vi "UART Write.vi"() -> ()   [LabVIEW 2023, in "CTI-Visa-Scratchpad.lvlib"]
uses:
  CTI-Visa-Scratchpad.lvlib
  CTI-Visa/CTI-Visa.lvlib
panel:
  in  "RX GPIO":u8=1
  in  "TX GPIO":u8
  in  "Baud":u32=19200
  in  "UART":u8
  in  "Write":bool
  in  "Data":string="Hello, world!"
  in  "stop":bool
  in  "Port":refnum<visa-resource-name>="COM3"
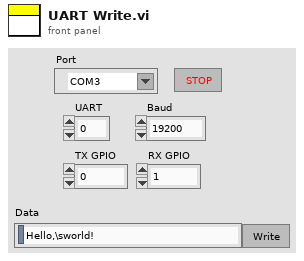
[diagram p1: front panel]
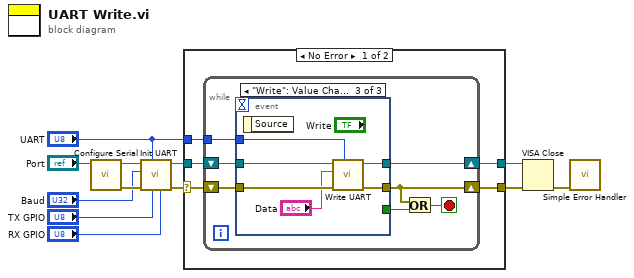
[diagram p0: block diagram]
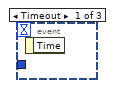
[diagram p2: hidden frame]
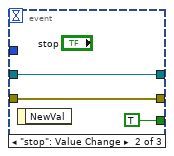
[diagram p3: hidden frame]
diagram:
  n1 = call "Configure Serial.vi"("VISA resource name in"="Port") -> ("error out"=w10:errorcluster, "VISA resource name"=w11:refnum<visa-resource-name>)  [unwired: 9 in]
  n2 = call "Init UART.vi"("RX GPIO"="RX GPIO", "TX GPIO"="TX GPIO", "UART"="UART", "error in (no error)"=w10, "Baud"="Baud", "VISA resource name in"=w11) -> ("error out"=w9:errorcluster, "VISA resource name"=w8:refnum<visa-resource-name>)  [unwired: 4 in]
  n3 = case shown="No Error" w9 {
    selector: w9 -> [w15 w35]
    tunnel: w8 -> [w16 w34]
    tunnel: "UART" -> [w17 _]
    tunnel: [w14 w35] -> w7
    tunnel: [w13 w34] -> w6
    frame No Error {
      n4 = while {
        tunnel: w17 -> [w23]
        shift-right: [w22] -> w13
        shift-left: w16 -> [w24]
        shift-right: [w20] -> w14
        shift-left: w15 -> [w21]
        stop <- w18 stop-if-true
        n5 = event shown="[2] \"Write\": Value Change" {
          selector: _ -> [_ _ _]
          dyn-events: _ -> [_ _ _]
          timeout: _ -> [_ _ _]
          tunnel: w24 -> [_ w27 w33]
          tunnel: w23 -> [_ _ w29]
          tunnel: [_ w27 w31] -> w22
          tunnel: w21 -> [_ w26 w32]
          tunnel: [_ w26 w30] -> w20
          tunnel: [_ TRUE _] -> w19
          event Timeout {
            n6 = event-data() -> ()  [unwired: 1 in, 1 out]
          }
          event "stop": Value Change {
            n7 = event-data() -> ()  [unwired: 1 in, 1 out]
          }
          event "Write": Value Change {
            n8 = event-data() -> ()  [unwired: 1 in, 1 out]
            n9 = call "Write UART.vi"("UART"=w29, "error in (no error)"=w32, "Data"="Data", "VISA resource name in"=w33) -> ("error out"=w30:errorcluster, "VISA resource name"=w31:refnum<visa-resource-name>)  [unwired: 6 in]
          }
        }
        n10 = Or(x=w20, y=w19) -> (x .or. y?=w18:bool)
      }
    }
    frame Error {
    }
  }
  n11 = VISA Close(VISA resource name=w6, error in (no error)=w7) -> (error out=w5:errorcluster)
  n12 = call <vilib>:"Simple Error Handler.vi"("error in (no error)"=w5) -> ()  [unwired: 4 in, 5 out]
